vi "LocateCorruptedSgmt.vi"(8 "error in":errorcluster, 11 "file path (use dialog)":path) -> (0 "error out":errorcluster, 2 "corrupted sgmt":i32, 3 "path":path)   [LabVIEW 2016]
panel:
  out "# of sgmts":i32
  out "NextSgmt Offsets Correct?":bool
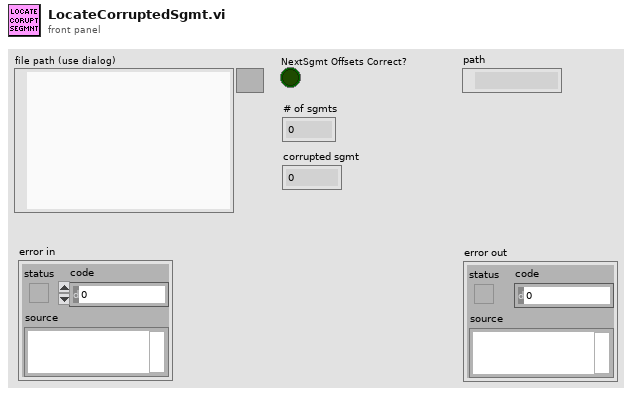
[diagram p1: front panel]
types:
  T1 = enum16{"open", "open or create", "create or replace", "create", "open (read-only)"}
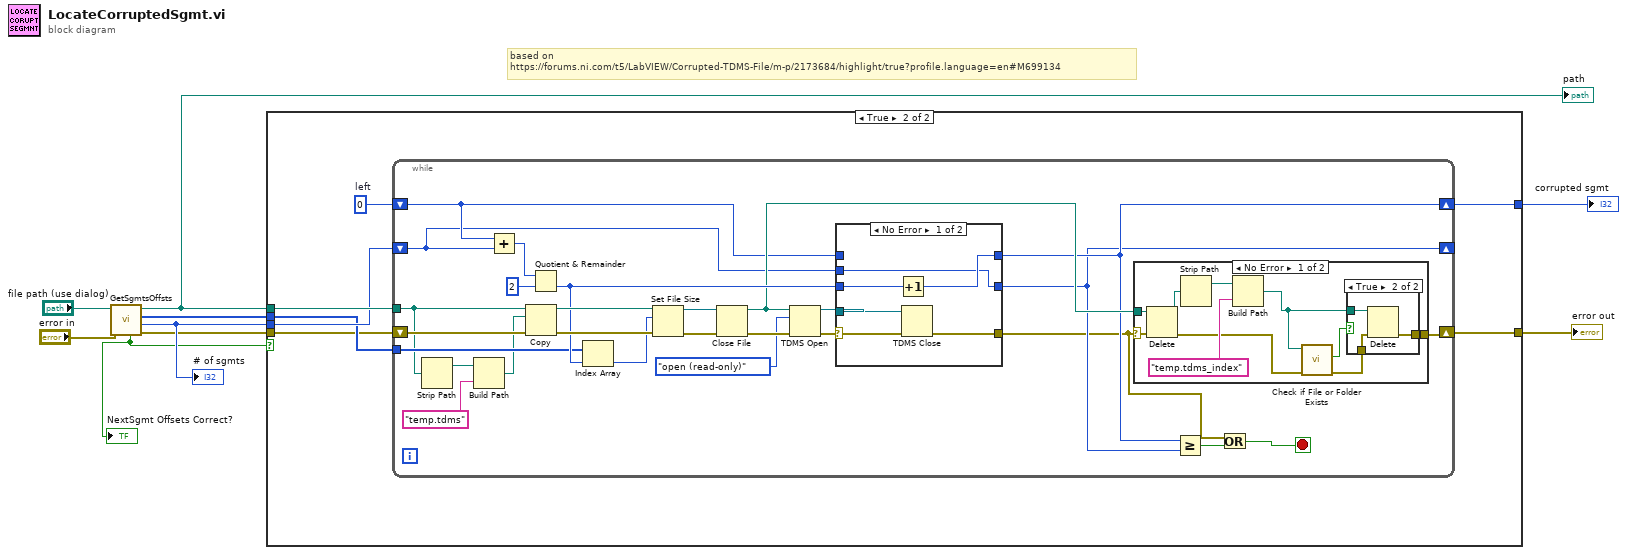
[diagram p0: block diagram]
diagram:
  # "based on\nhttps://forums.ni.com/t5/LabVIEW/Corrupted-TDMS-File/m-p/2173684/highlight/true?profile.language=en#M699134"
  n1 = call "GetSgmtsOffsts.vi"("error in"="error in", "file path (use dialog)"="file path (use dialog)") -> ("error out"=w7:errorcluster, "# of sgmts"=w8:i32, "offsets"=w3:u64[], "path"=w2:path, "Pass?"=w5:bool)  [unwired: 5 in]
  "NextSgmt Offsets Correct?" <- w5
  "# of sgmts" <- w8
  "path" <- w2
  n2 = case shown="True" w5 {
    tunnel: w2 -> [_ w17]
    tunnel: w8 -> [w10 w16]
    tunnel: w3 -> [_ w15]
    tunnel: w7 -> [w11 w14]
    tunnel: [w11 w13] -> w6
    tunnel: [w10 w12] -> w4
    frame False {
    }
    frame True {
      w18 = 0  # left
      n3 = while {
        shift-right: [w22] -> w12
        shift-left: w18 -> [w24]
        shift-right: [w21] -> _
        shift-left: w16 -> [w23]
        tunnel: w17 -> [w27]
        tunnel: w15 -> [w34]
        shift-right: [w25] -> w13
        shift-left: w14 -> [w32]
        stop <- w20 stop-if-true
        n4 = Strip Path(path=w27) -> (stripped path=w30:path)  [unwired: 1 out]
        n5 = Build Path(base path=w30, name or relative path="temp.tdms") -> (appended path=w28:path)
        n6 = Add(x=w24, y=w23) -> (x+y=w43:i32)
        n7 = Copy(8:w32, 10:w28, 11:w27) -> (0:w44:errorcluster, 3:w45:path)  [unwired: 2 in, 1 out]
        n8 = Quotient & Remainder(x=w43, y=2) -> (floor(x/y)=w35:i32)  [unwired: 1 out]
        n9 = Index Array(array=w34, index=w35) -> (element=w33:u64)
        n10 = Set File Size(4:w44, 6:w33, 7:w45) -> (0:w40:errorcluster, 3:w41:refnum<file>)
        n11 = Close File(refnum=w41, error in=w40) -> (path=w26:path, error out=w39:errorcluster)
        n12 = TDMS Open(8:w39, 10:T1."open (read-only)" ("operation (0:open)"), 11:w26) -> (0:w37:errorcluster, 3:w36:refnum<k34>)  [unwired: 4 in]
        n13 = case shown="No Error" w37 {
          selector: w37 -> [w64 w67]
          tunnel: w35 -> [w66 w68]
          tunnel: [w61 w68] -> w21
          tunnel: [w63 w67] -> w19
          tunnel: w36 -> [w62 _]
          tunnel: w24 -> [_ w69]
          tunnel: w23 -> [w61 _]
          tunnel: [w65 w69] -> w22
          frame No Error {
            n14 = Increment(x=w66) -> (x+1=w65:i32)
            n15 = TDMS Close(8:w64, 11:w62) -> (0:w63:errorcluster)  [unwired: 1 out]
          }
          frame Error {
          }
        }
        n16 = case shown="No Error" w19 {
          selector: w19 -> [w46 w60]
          tunnel: w26 -> [w55 _]
          tunnel: [w54 w60] -> w25
          frame No Error {
            n17 = Delete(path (use dialog)=w55, error in=w46) -> (deleted path=w53:path, error out=w50:errorcluster)  [unwired: 3 in, 1 out]
            n18 = Strip Path(path=w53) -> (stripped path=w52:path)  [unwired: 1 out]
            n19 = Build Path(base path=w52, name or relative path="temp.tdms_index") -> (appended path=w49:path)
            n20 = call <vilib>:"Check if File or Folder Exists.vi"("error in (no error)"=w50, "path"=w49) -> ("error out"=w47:errorcluster, "file or folder exists?"=w48:bool)  [unwired: 7 in, 1 out]
            n21 = case shown="True" w48 {
              tunnel: [w56 w59] -> w54
              tunnel: w49 -> [_ w58]
              tunnel: w47 -> [w56 w57]
              frame False {
              }
              frame True {
                n22 = Delete(path (use dialog)=w58, error in=w57) -> (error out=w59:errorcluster)  [unwired: 3 in, 2 out]
              }
            }
          }
          frame Error {
          }
        }
        n23 = Greater Or Equal?(x=w22, y=w21) -> (x >= y?=w31:bool)
        n24 = Or(x=w19, y=w31) -> (x .or. y?=w20:bool)
      }
    }
  }
  "error out" <- w6
  "corrupted sgmt" <- w4
